vi "ts_tree_set_column_1_data.vi"(8 "error in (no error)":errorcluster, 9 "String":string, 10 "ts.data":T1, 11 "test.results.ref":refnum<vi>) -> (0 "error out":errorcluster)   [LabVIEW 2015]
uses:
  ts-data.ctl
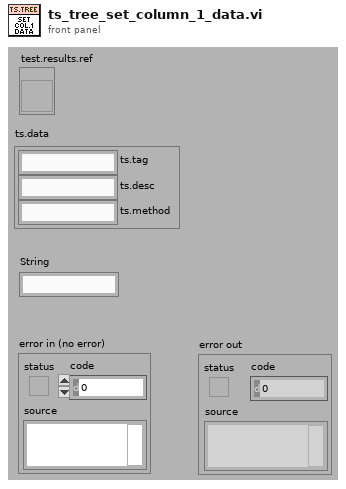
[diagram p1: front panel]
types:
  T1 = typedef "ts-data.ctl" = cluster{"ts.tag":string, "ts.desc":string, "ts.method":string}
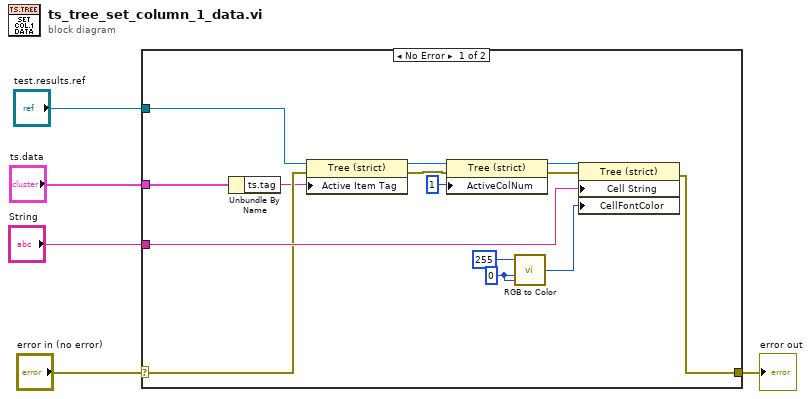
[diagram p0: block diagram]
diagram:
  n1 = case shown="No Error" "error in (no error)" {
    selector: "error in (no error)" -> [w10 w20]
    tunnel: [w9 w20] -> w4
    tunnel: "String" -> [w14 _]
    tunnel: "ts.data" -> [w8 _]
    tunnel: "test.results.ref" -> [w6 _]
    frame No Error {
      w17 = u8 0 ("G")
      n2 = Unbundle By Name(w8) -> ("ts.tag"=w7:string)
      n3 = property class="Tree (strict)"(reference=w6, error in=w10, "Active Item Tag"=w7) -> (reference out=w13:refnum<vi>, error out=w12:errorcluster)
      n4 = property class="Tree (strict)"(reference=w13, error in=w12, "ActiveColNum"=1 ("Active Cell:Active Column Number")) -> (reference out=w19:refnum<vi>, error out=w11:errorcluster)
      n5 = call <vilib>:"RGB to Color.vi"("B"=w17, "G"=w17, "R"=u8 255) -> ("Color"=w16:u32)
      n6 = property class="Tree (strict)"(reference=w19, error in=w11, "Cell String"=w14, "CellFontColor"=w16) -> (error out=w9:errorcluster)  [unwired: 1 out]
    }
    frame Error {
    }
  }
  "error out" <- w4
